vi "FitXYCenterData.vi"(4 "True  data <-> Simulation\nOff: True data\nOn: Simulated data":bool, 5 "Fit Method":u16(ring) items=["WLC (Default)", "Symmetry", "1st and 3rd order Func Fit", "Symmetry (Older version)"], 6 "Cluster":T1={"offset Xsignal [pN]"=20.0, "offset PX [nm]"=100.0, "offset PY [nm]"=100.0, "kBT"=4.1, "Noise lvl [pN]"=0.2, "Contour length [nm]"=2000.0, "Persistence length [nm]"=40.0, "step length [nm]"=10.0, "Total scan range [nm]"=2500.0, "trap height [nm]"=1000.0}, 7 "Data input":cluster{dbl[], dbl[]}) -> (0 "The methods have been used":string, 1 "Parameters":cluster{"PX center":dbl, "Xsignal Baseline":dbl}, 2 "Residues":cluster{"X converted":dbl[], "Residue":dbl[]}(graph), 3 "data and fit":cluster{dbl[], "Best Polynomial Fit":dbl[]}[](graph))   [LabVIEW 2020, in "XYcenter.lvlib"]
uses:
  XYcenter.lvlib
  <vilib>/Analysis/baseanly.llb/Unimode.vi
  <vilib>/gmath/NumericalOptimization/Nonlinear Curve Fit LM.vi
  <vilib>/gmath/NI_Gmath.lvlib
  <vilib>/Analysis/NI_AALPro.lvlib
  <vilib>/Analysis/NI_AALBase.lvlib
  BasicVIs/BasicVIs.lvlib
panel:
  in  "points to average":i32=3
  in  "termination":cluster{"max iteration":i32, "tolerance":dbl}={"max iteration"=200, "tolerance"=1e-08}
  out "number of function calls":i32
  out "monotonically increase?":bool
  out "Guesses":dbl[](array[numeric])
  out "error out":errorcluster
  out "best fit parameters:\nPX center, Xsignal Baseline, 1th and 3rd order coeffs":dbl[](array[numeric])
  # "X0, Y0, A0, L0"
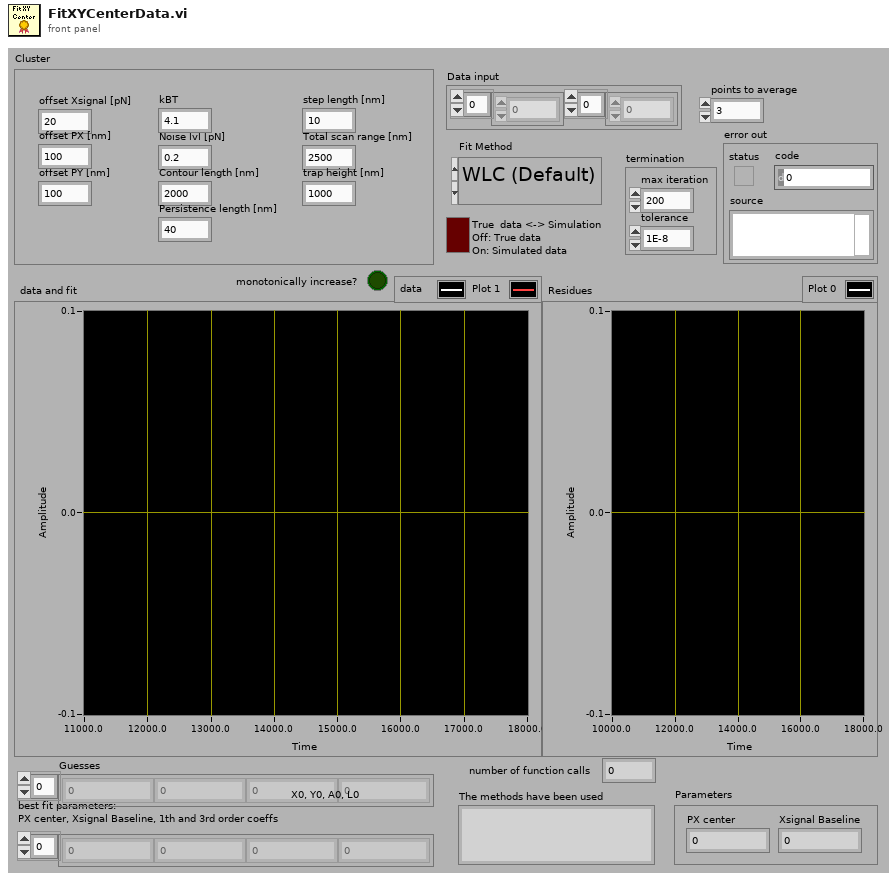
[diagram p1: front panel]
types:
  T1 = cluster{"offset Xsignal [pN]":dbl, "offset PX [nm]":dbl, "offset PY [nm]":dbl, "kBT":dbl, "Noise lvl [pN]":dbl, "Contour length [nm]":dbl, "Persistence length [nm]":dbl, "step length [nm]":dbl, "Total scan range [nm]":dbl, "trap height [nm]":dbl}
  T2 = cluster{"X converted":dbl[], "Y converted":dbl[]}
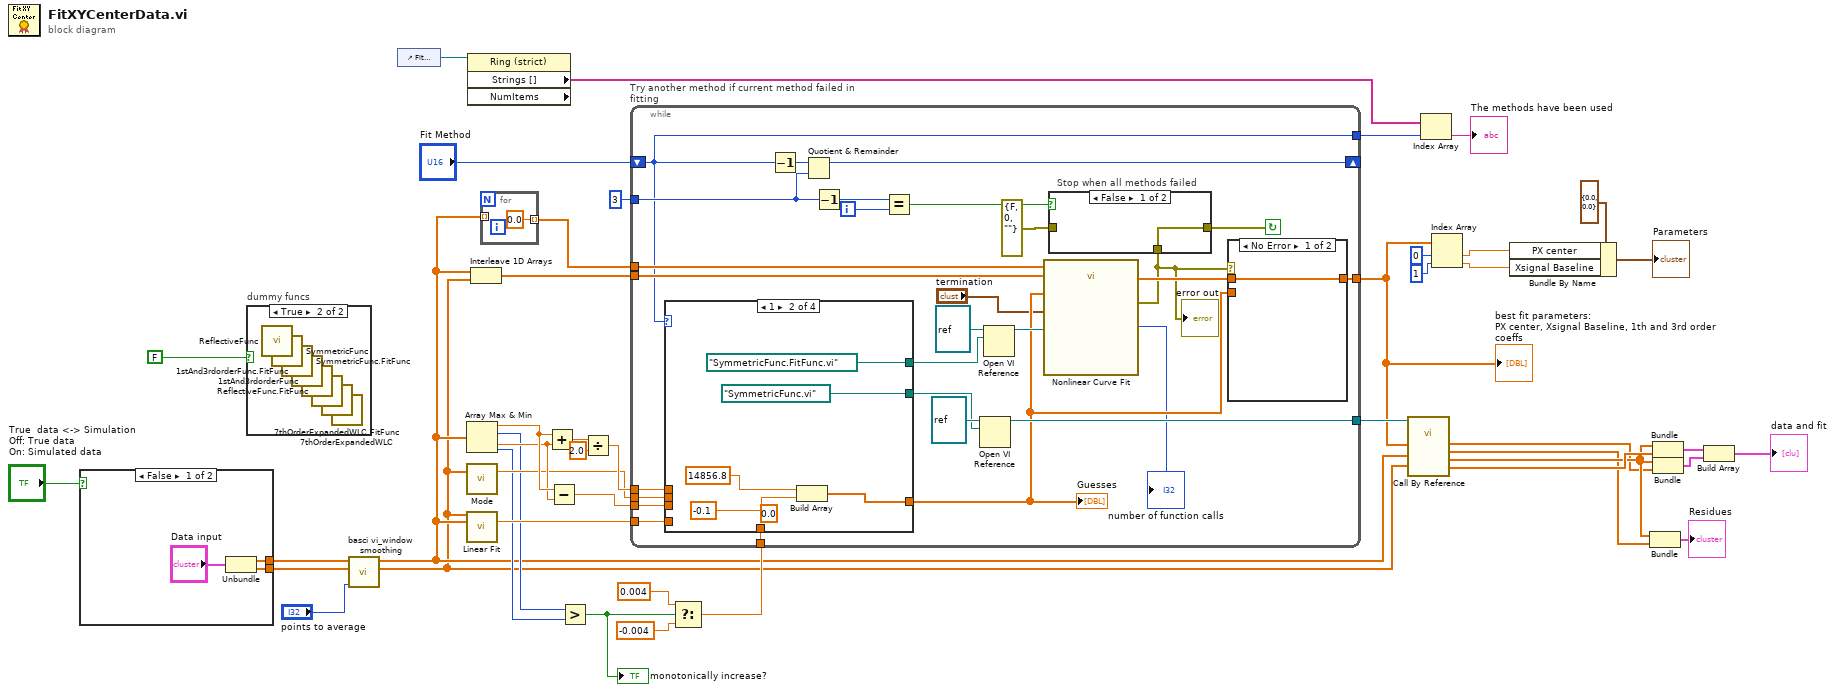
[diagram p0: block diagram]
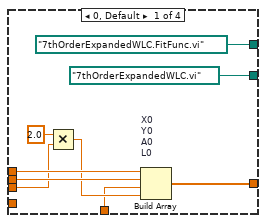
[diagram p5: hidden frame]
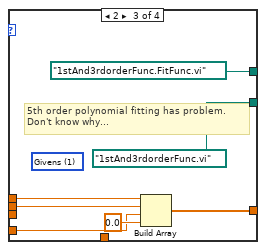
[diagram p6: hidden frame]
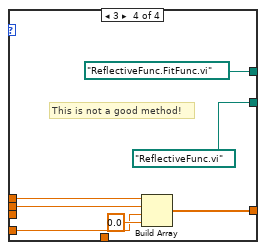
[diagram p7: hidden frame]
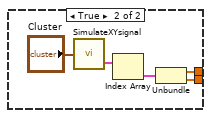
[diagram p8: hidden frame]
diagram:
  n1 = case shown="False" "True  data <-> Simulation\nOff: True data\nOn: Simulated data" {
    tunnel: [w48 w50] -> w7
    tunnel: [w47 w49] -> w6
    frame False {
      n2 = Unbundle("Data input") -> (w48:dbl[], w47:dbl[])
    }
    frame True {
      n3 = call "SimulateXYsignal.vi"("Cluster"="Cluster") -> ("XY Graph"=w52:cluster{dbl[], dbl[]}[])  [unwired: 1 out]
      n4 = Index Array(array=w52) -> (element=w51:cluster{dbl[], dbl[]})  [unwired: 1 in]
      n5 = Unbundle(w51) -> (w50:dbl[], w49:dbl[])
    }
  }
  n6 = case "dummy funcs" shown="True" FALSE {
    frame False {
    }
    frame True {
      n7 = call "ReflectiveFunc.vi"() -> ()  [unwired: 3 in, 4 out]
      n8 = call "SymmetricFunc.vi"() -> ()  [unwired: 3 in, 4 out]
      n9 = call "SymmetricFunc.FitFunc.vi"() -> ()  [unwired: 4 in, 3 out]
      n10 = call "1stAnd3rdorderFunc.FitFunc.vi"() -> ()  [unwired: 4 in, 3 out]
      n11 = call "1stAnd3rdorderFunc.vi"() -> ()  [unwired: 3 in, 4 out]
      n12 = call "ReflectiveFunc.FitFunc.vi"() -> ()  [unwired: 4 in, 3 out]
      n13 = call "7thOrderExpandedWLC.FitFunc.vi"() -> ()  [unwired: 4 in, 3 out]
      n14 = call "7thOrderExpandedWLC.vi"() -> ()  [unwired: 3 in, 4 out]
    }
  }
  n15 = call "basci vi_window smoothing.vi"("points to average"="points to average", "Y"=w6, "X"=w7) -> ("Y smoothed"=w4:dbl[], "X smoothed"=w5:dbl[])  [unwired: 3 in]
  n16 = control-ref of="Fit Method"() -> (w28:refnum<vi>)
  n17 = Array Max & Min(array=w5) -> (max value=w18:dbl, max index (indices)=w13:i32, min value=w17:dbl, min index (indices)=w12:i32)
  n18 = call-poly <vilib>:"Mode.vi"("X"=w4) -> ("mode"=w14:dbl)  [unwired: 1 in, 1 out]
  n19 = call <vilib>:"Linear Fit.vi"("Y"=w4, "X"=w5) -> ("slope"=w23:dbl)  [unwired: 9 in, 4 out]
  n20 = property on="属性节点" class="Ring (strict)" props=["Strings []", "NumItems"](reference=w28) -> ("Strings []"=w26:string[])  [unwired: 1 in, 3 out]
  n21 = Interleave 1D Arrays(w5, w4) -> (w45:dbl[])
  n22 = for {
    tunnel: w5 -> [_] mode=indexing
    tunnel: [0.0] -> w41 mode=indexing
  }
  n23 = Add(x=w18, y=w17) -> (x+y=w44:dbl)
  n24 = Subtract(x=w18, y=w17) -> (x-y=w16:dbl)
  n25 = Greater?(x=w13, y=w12) -> (0:w10:bool)
  "monotonically increase?" <- w10
  n26 = Divide(x=w44, y=2.0) -> (x/y=w15:dbl)
  n27 = Select(t=0.004 ("element"), s=w10, f=-0.004 ("element")) -> (s? t:f=w8:dbl)
  n28 = while "Try another method if current method failed in fitting" {
    tunnel: w45 -> [w80]
    tunnel: w15 -> [w79]
    tunnel: w14 -> [w78]
    tunnel: [w74] -> w42
    tunnel: w41 -> [w73]
    tunnel: [w69] -> w33
    shift-right: [w64] -> _
    shift-left: "Fit Method" -> [w63]
    tunnel: u32 3 ("NumItems") -> [w67]
    tunnel: [w63] -> w24
    tunnel: w23 -> [w62]
    tunnel: w16 -> [w60]
    tunnel: w8 -> [w57]
    i -> [w71]
    stop <- w55 continue-if-true
    n29 = case shown="1" w63 {
      tunnel: [path "7thOrderExpandedWLC.FitFunc.vi" path "SymmetricFunc.FitFunc.vi" path "1stAnd3rdorderFunc.FitFunc.vi" path "ReflectiveFunc.FitFunc.vi" ("vi path")] -> w81
      tunnel: w79 -> [w92 _ w103 w113]
      tunnel: [w94 w99 w106 w112] -> w68
      tunnel: w78 -> [w91 _ w102 w111]
      tunnel: [path "7thOrderExpandedWLC.vi" path "SymmetricFunc.vi" path "1stAnd3rdorderFunc.vi" path "ReflectiveFunc.vi" ("vi path")] -> w75
      tunnel: w62 -> [_ _ w101 w108]
      tunnel: w60 -> [w90 _ _ _]
      tunnel: w57 -> [w87 _ _ _]
      frame 0, Default {
        n30 = Multiply(x=2.0, y=w90) -> (x*y=w88:dbl)
        n31 = Build Array "X0\nY0\nA0\nL0"(w92, w91, w87, w88) -> (w94:dbl[])
      }
      frame 1 {
        (unwired) 0.0 ("element")
        n32 = Build Array(14856.8, -0.1) -> (w99:dbl[])
      }
      frame 2 {
        (unwired) u16 1 items=["SVD", "Givens", "Givens2", "Householder", "LU分解", "Cholesky", "不满秩H的SVD"] ("algorithm")
        # "5th order polynomial fitting has problem. \nDon't know why..."
        n33 = Build Array(w103, w102, w101, 0.0 ("element")) -> (w106:dbl[])
      }
      frame 3 {
        # "This is not a good method!"
        n34 = Build Array(w113, w111, w108, 0.0 ("element")) -> (w112:dbl[])
      }
    }
    "Guesses" <- w68
    n35 = Decrement(x=w63) -> (x-1=w65:u32)
    n36 = Quotient & Remainder(x=w65, y=w67) -> (x-y*floor(x/y)=w64:u32)  [unwired: 1 out]
    n37 = Decrement(x=w67) -> (x-1=w66:u32)
    n38 = Equal?(x=w66, y=w71) -> (x = y?=w72:bool)
    n39 = Open VI Reference(type specifier VI Refnum (for type only)=refnum<vi> refnum, vi path=w75) -> (vi reference=w74:refnum<vi>)  [unwired: 4 in, 1 out]
    n40 = Open VI Reference(type specifier VI Refnum (for type only)=refnum<vi> refnum, vi path=w81) -> (vi reference=w77:refnum<vi>)  [unwired: 4 in, 1 out]
    n41 = call-poly <vilib>:"Nonlinear Curve Fit.vi"("Y"=w73, "f(x,a)"=w77, "X"=w80, "initial parameters"=w68, "termination"="termination") -> ("number of function calls"=→"number of function calls":i32, "best fit parameters"=w70:dbl[], "error out"=w58:errorcluster)  [unwired: 5 in, 3 out]
    "error out" <- w58
    n42 = case "Stop when all methods failed" shown="False" w72 {
      tunnel: w58 -> [w85 _]
      tunnel: [w85 w86] -> w55
      tunnel: errorcluster {"status"=FALSE, "code"=0, "source"=""} ("error out") -> [_ w86]
      frame False {
      }
      frame True {
      }
    }
    n43 = case shown="No Error" w58 {
      tunnel: w70 -> [w83 _]
      tunnel: [w83 w84] -> w69
      tunnel: w68 -> [_ w84]
      frame No Error {
      }
      frame Error {
        # "If All methods\nFailed, return \ninitial guess"
      }
    }
  }
  "best fit parameters:\nPX center, Xsignal Baseline, 1th and 3rd order coeffs" <- w33
  n44 = call-by-ref "?"(reference=w42, "Y"=w4, "X"=w5, "Coefficients"=w33) -> ("Y converted"=w37:dbl[], "X converted"=w35:dbl[], "Residue"=w34:dbl[], "f(X,a)"=w2:dbl[])  [unwired: 1 in, 2 out]
  n45 = Index Array(array=w26, index=w24) -> (element=→"The methods have been used":string)
  n46 = Index Array(array=w33, index #1=0 ("index"), index #2=1 ("index")) -> (element #1=w22:dbl, element #2=w21:dbl)
  n47 = Bundle By Name(cluster=cluster{"PX center":dbl, "Xsignal Baseline":dbl} {"PX center"=0.0, "Xsignal Baseline"=0.0} ("Parameters"), "PX center"=w22, "Xsignal Baseline"=w21) -> (→"Parameters":cluster{"PX center":dbl, "Xsignal Baseline":dbl})
  n48 = Bundle("X converted"=w35, "Residue"=w34) -> (→"Residues":cluster{"X converted":dbl[], "Residue":dbl[]})  [unwired: 1 in]
  n49 = Bundle("X converted"=w35, "Y converted"=w37) -> (w40:T2)  [unwired: 1 in]
  n50 = Bundle("X converted"=w35, "f(X,a)"=w2) -> (w39:cluster{"X converted":dbl[], "f(X,a)":dbl[]})  [unwired: 1 in]
  n51 = Build Array(w40, w39) -> (→"data and fit":cluster{"X converted":dbl[], "f(X,a)":dbl[]}[])
